vi "PH_PSDBController.ProcCases.vi"(0 "i ref in":refnum<vi>, 1 "selector":string, 2 "Data":T1, 3 "call cluster":T2={"Object"="", "Selector"="", "CallType"=enum."synchronous", "Async Object"="", "Async Selector"="", "Data Descriptor"="", "Data"=[], "Error #"=0, "Expire"=0}, 5 "error in":errorcluster) -> (14 "i ref out":refnum<vi>, 17 "answer cluster":T2={"Object"="", "Selector"="", "CallType"=enum."synchronous", "Async Object"="", "Async Selector"="", "Data Descriptor"="", "Data"=[], "Error #"=0, "Expire"=0}, 19 "error out":errorcluster)   [LabVIEW 2014, in "PH_PSDBController.lvlib"]
doc: "This method is called by a process from within the default case in the event loop. The methods of a class that are linked to events will be called from THIS method. Add your code here."
uses:
  PH_PSDBController.lvlib
  CSCore/CSSystem/CoreDefs/CoreDefs.call_type.ctl
  CSCore/BaseProcess/BaseProcess.descriptor string definition.ctl
  CSCore/CSSystem/CoreDefs/CoreDefs.rawDataType.ctl
  PH_PSDBWriter/PH_PSDBWriter.Data Status.ctl
  PH_Beamline_Chief/PH_Beamline_Chief.Section.ctl
  PH_PSDBWriter/PH_PSDBWriter.PHELIX-Subsystems.ctl
  CSCore/CSSystem/CoreLib/CoreLib.string 2 byte array.vi
  CSCore/CSSystem/CoreLib/CoreLib.byte array 2 short.vi
  CSCore/CSSystem/CoreLib/CoreLib.byte array 2 string.vi
  CSCore/BaseProcess/BaseProcess.lvlib
  CSCore/CSSystem/CoreLib/CoreLib.lvlib
  CSCore/CAEObj/CAEObj.lvlib
  PH_PSDBWriter/PH_PSDBWriter.lvlib
  PH_Common/PH_Common.lvlib
  lib.lib/DimLVEvent/LVDimInterface/LVDimInterface.lvlib
  lib.lib/UtilityLib/UtilityLib.lvlib
  PH_Beamline_Chief/PH_Beamline_Chief.lvlib
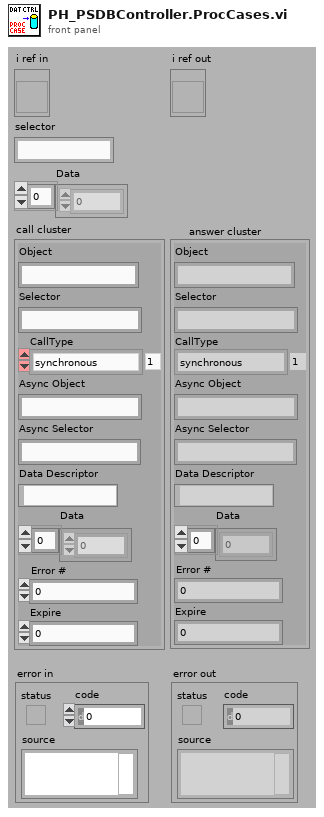
[diagram p1: front panel]
types:
  T1 = typedef "CoreDefs.rawDataType.ctl" = i8[]
  T2 = typedef "CoreDefs.call_type.ctl" = cluster{"Object":string, "Selector":string, "CallType":enum16{"simple", "synchronous", "asynchronous"}, "Async Object":string, "Async Selector":string, "Data Descriptor":T3, "Data":T1, "Error #":i32, "Expire":u32}
  T3 = typedef "BaseProcess.lvlib/BaseProcess.descriptor string definition.ctl" = string
  T4 = typedef "PH_PSDBWriter.lvlib/PH_PSDBWriter.Data Status.ctl" = i16
  T5 = typedef "PH_PSDBController.lvlib/PH_PSDBController.i attribute.ctl" = cluster{"GUI Refs":cluster{"Data Status":refnum<vi>, "Current Shot ID":refnum<vi>, "active Subsystems":refnum<vi>, "Experiment Description":refnum<vi>, "Shot Comment":refnum<vi>, "Experiment":refnum<vi>, "Shottype":refnum<vi>, "Sequencer SM State":refnum<vi>, "Instances with Errors":refnum<vi>}, "Service ID Shot ID":i32, "Service ID wanted Subsystem":i32, "Data Status":T4, "Shotinformation":cluster{"Current Experiment ID":i32, "Current Shot Type":i32, "Current Comment":string}, "Data taking?":bool, "Service ID current Shottype":i32, "Service ID current Experiment":i32, "Service ID currentShot Comment":i32, "Service ID possible Shottypes":i32, "Service ID possible Experiments":i32, "possible Experiments":T6[], "possible Shottypes":T6[], "List":cluster{"Info":cluster{"Instance":string, "Data Status":T4}[], "GUI Ref":refnum<vi>, "Classname":string}[], "Subsystems Off?":cluster{"PHELIX_Beamline_fs_YLF_BL_Status":bool, "PHELIX_Beamline_ns_BL_Status":bool, "PHELIX_Beamline_PA_Input_BL_Status":bool, "PHELIX_Beamline_PA_MA_BL_Status":bool, "PHELIX_Beamline_MA_Z6_BL_Status":bool, "PHELIX_Beamline_MA_LB_BL_Status":bool, "PHELIX_Beamline_PA_LL_BL_Status":bool}, "PSDB Credentials":T7}
  T6 = typedef "PSDB.lvlib/PSDB_Info.ctl" = cluster{"Name":string, "Description":string, "ID":i32}
  T7 = typedef "PH_Common.lvlib/PH_Connection.PSDB Credentials.ctl" = cluster{"PW":string, "ID":string, "DS":string}
  T8 = typedef "PH_Beamline_Chief.lvlib/PH_Beamline_Chief.Section.ctl" = enum16{"None", "YLF", "fs", "fs-YLF", "ns", "PA-Input", "PA-Undelay", "PA-Delay", "PA-before-Bypass", "PA", "PA-Bypass", "PA-Exit", "PA-LL", "LL", "PA-MA", "MA-Exit", "MA-Z6", "Z6", "MA-LB", "LB-TB2", "LB-TB3"}
  T9 = typedef "PH_PSDBWriter.lvlib/PH_PSDBWriter.PHELIX-Subsystems.ctl" = i32
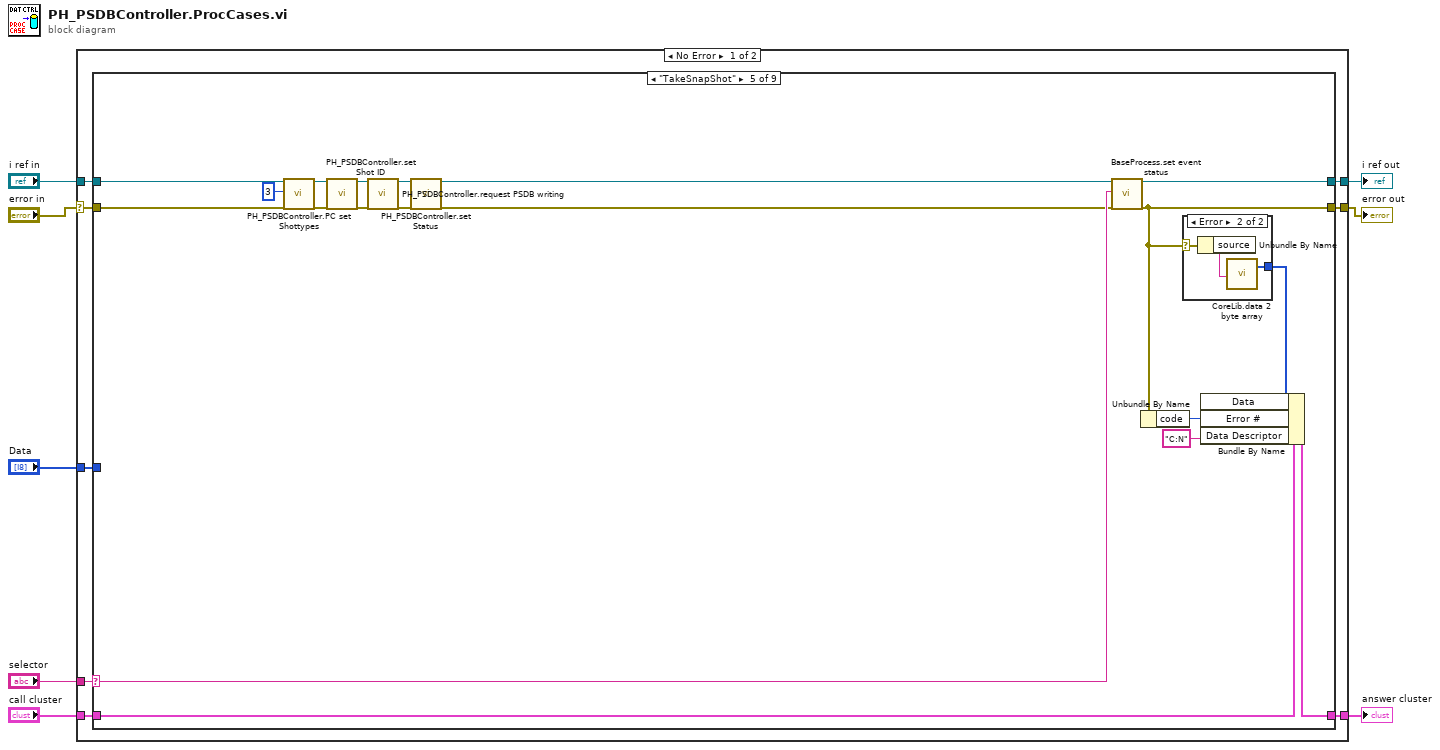
[diagram p0: block diagram]
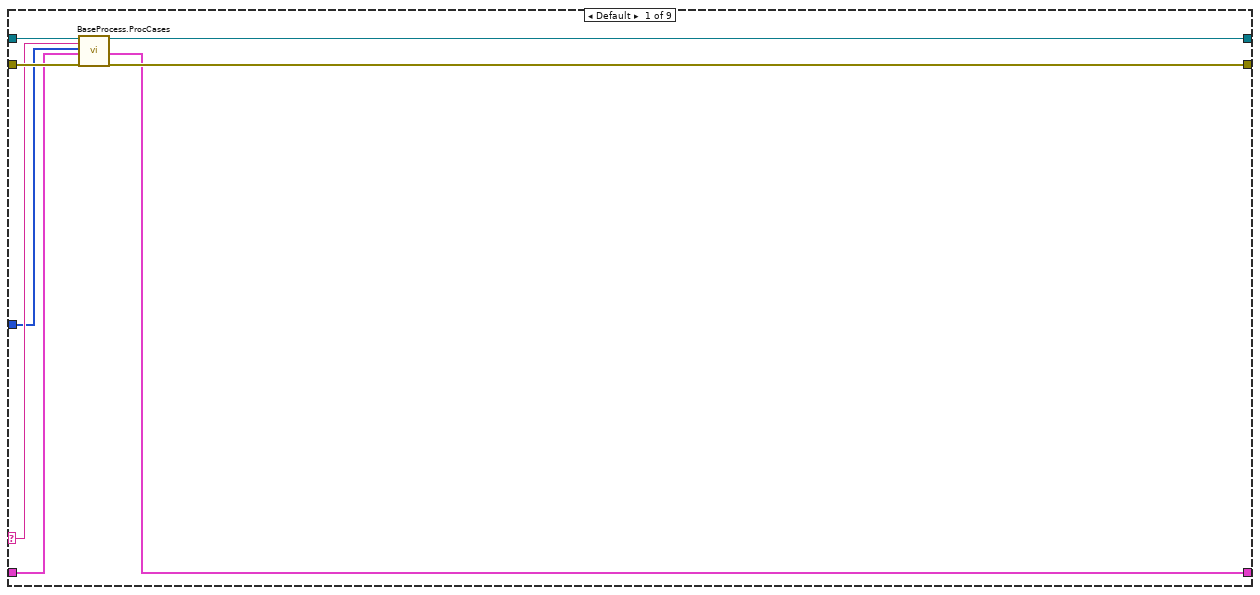
[diagram p2: hidden frame]
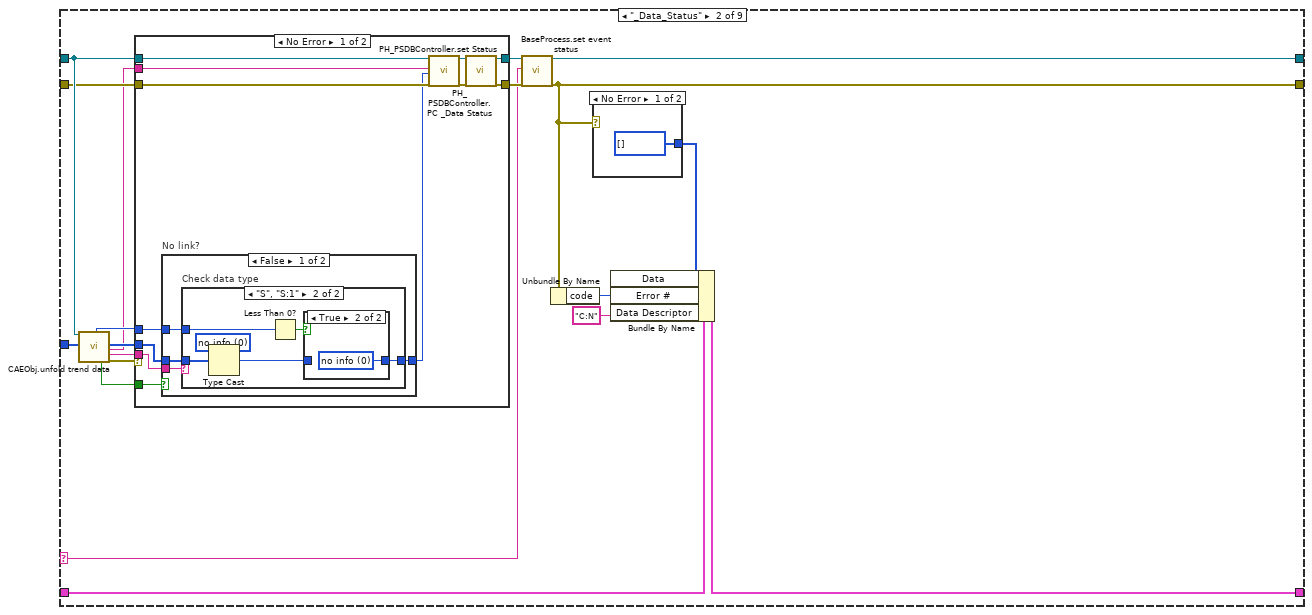
[diagram p3: hidden frame]
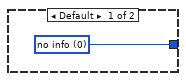
[diagram p4: hidden frame]
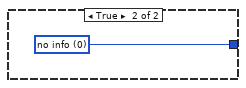
[diagram p6: hidden frame]
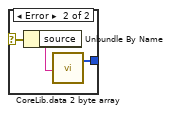
[diagram p8: hidden frame]
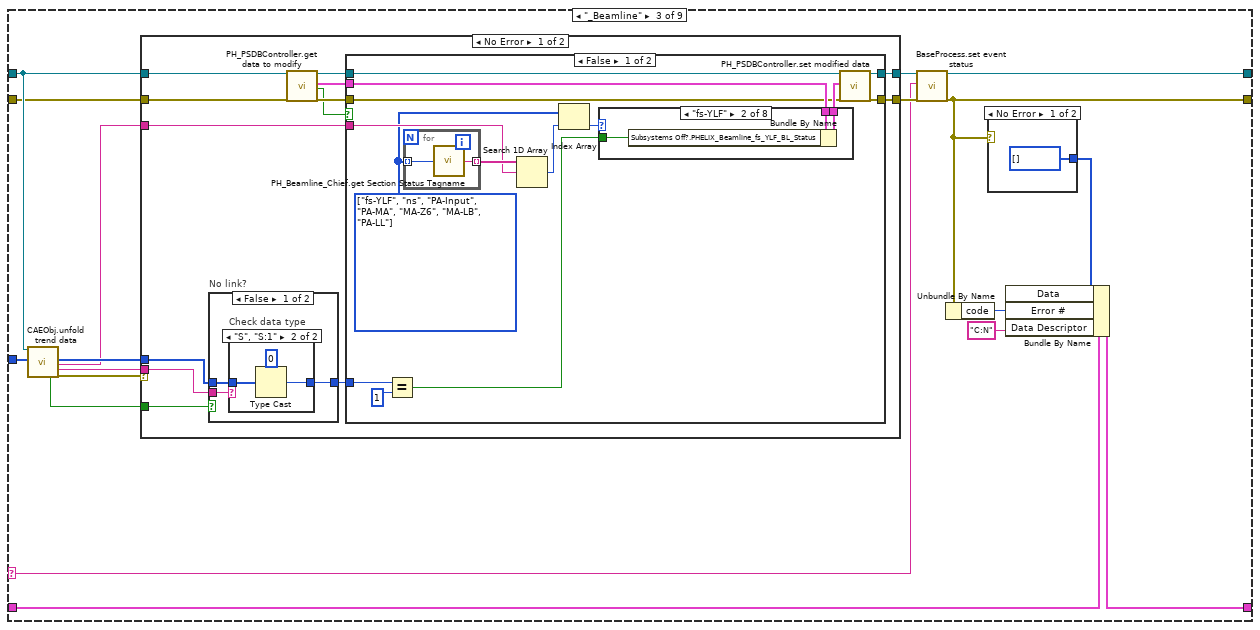
[diagram p9: hidden frame]
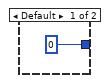
[diagram p10: hidden frame]
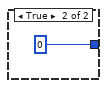
[diagram p11: hidden frame]
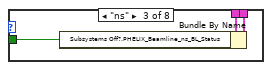
[diagram p13: hidden frame]
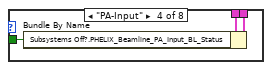
[diagram p14: hidden frame]
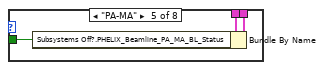
[diagram p15: hidden frame]
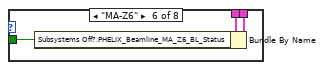
[diagram p16: hidden frame]
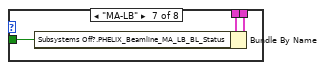
[diagram p17: hidden frame]
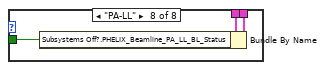
[diagram p18: hidden frame]
diagram:
  n1 = case shown="No Error" "error in" {
    selector: "error in" -> [w9 w435]
    tunnel: "selector" -> [w16 _]
    tunnel: [w15 w434] -> w7
    tunnel: "call cluster" -> [w14 w434]
    tunnel: "i ref in" -> [w13 w436]
    tunnel: [w12 w436] -> w4
    tunnel: [w11 w435] -> w3
    tunnel: "Data" -> [w10 _]
    frame No Error {
      n2 = case shown="\"TakeSnapShot\"" w16 {
        selector: w16 -> [w19 w33 w87 w168 w294 w302 w332 w366 w380]
        tunnel: w10 -> [w17 w26 w80 w161 _ _ _ _ _]
        tunnel: w13 -> [w18 w32 w86 w167 w280 w309 w339 w368 w387]
        tunnel: [w24 w31 w85 w166 w293 w313 w343 w372 w391] -> w12
        tunnel: w14 -> [w20 w28 w82 w163 w290 w306 w336 w367 w384]
        tunnel: [w21 w29 w83 w164 w291 w311 w341 w370 w389] -> w15
        tunnel: w9 -> [w23 w27 w81 w162 w279 w310 w340 w369 w388]
        tunnel: [w22 w30 w84 w165 w292 w312 w342 w371 w390] -> w11
        frame Default {
          n3 = call "BaseProcess.ProcCases.vi"("i ref in"=w18, "selector"=w19, "Data"=w17, "call cluster"=w20, "error in (no error)"=w23) -> ("i ref out"=w24:refnum<vi>, "answer cluster"=w21:T2, "error out"=w22:errorcluster)  [unwired: 12 in]
        }
        frame "_Data_Status" {
          n4 = call "CAEObj.unfold trend data.vi"("i ref in"=w32, "raw trend data"=w26) -> ("quality"=w34:i32, "no link"=w37:bool, "data"=w35:i8[], "serviceName"=w25:string, "typeDescriptor"=w36:string, "error out"=w38:errorcluster)  [unwired: 9 in, 3 out]
          n5 = case shown="No Error" w38 {
            tunnel: w27 -> [w54 w71]
            tunnel: [w46 w70] -> w40
            tunnel: [w44 w71] -> w39
            tunnel: w32 -> [w55 w70]
            tunnel: w37 -> [w51 _]
            tunnel: w36 -> [w52 _]
            tunnel: w35 -> [w50 _]
            tunnel: w34 -> [w49 _]
            tunnel: w25 -> [w53 _]
            frame No Error {
              n6 = case "No link?" shown="False" w51 {
                tunnel: [w59 w69] -> w48
                tunnel: w49 -> [w58 _]
                tunnel: w50 -> [w57 _]
                tunnel: w52 -> [w56 _]
                frame False {
                  n7 = case "Check data type" shown="\"S\", \"S:1\"" w56 {
                    tunnel: [w60 w66] -> w59
                    tunnel: w58 -> [_ w64]
                    tunnel: w57 -> [_ w63]
                    frame Default {
                      w60 = T4 0 items=["no info", "no Data collection", "no problem", "Error getting the instance ID", "Error writing Data to data base", "Error concerning the subsystem"] ("Data Status")
                    }
                    frame "S", "S:1" {
                      w61 = T4 0 items=["no info", "no Data collection", "no problem", "Error getting the instance ID", "Error writing Data to data base", "Error concerning the subsystem"] ("Data Status")
                      n8 = Type Cast(type=w61, x=w63) -> (*(type *) &x=w62:T4)
                      n9 = Less Than 0?(x=w64) -> (x < 0?=w65:bool)
                      n10 = case shown="True" w65 {
                        tunnel: [w67 w68] -> w66
                        tunnel: w62 -> [w67 _]
                        frame False {
                        }
                        frame True {
                          w68 = T4 0 items=["no info", "no Data collection", "no problem", "Error getting the instance ID", "Error writing Data to data base", "Error concerning the subsystem"] ("Data Status")
                        }
                      }
                    }
                  }
                }
                frame True {
                  w69 = T4 0 items=["no info", "no Data collection", "no problem", "Error getting the instance ID", "Error writing Data to data base", "Error concerning the subsystem"] ("Data Status")
                }
              }
              n11 = call "PH_PSDBController.PC _Data Status.vi"("i ref in"=w55, "Data Status service name"=w53, "Data Status"=w48, "error IO"=w54) -> ("i ref out"=w47:refnum<vi>, "error out"=w45:errorcluster)  [unwired: 14 in]
              n12 = call "PH_PSDBController.set Status.vi"("i ref in"=w47, "error in"=w45) -> ("i ref out"=w46:refnum<vi>, "error out"=w44:errorcluster)  [unwired: 16 in]
            }
            frame Error {
            }
          }
          n13 = call "BaseProcess.set event status.vi"("i ref in"=w40, "EventStatus"=w33, "error in (no error)"=w39) -> ("i ref out"=w31:refnum<vi>, "error out"=w30:errorcluster)  [unwired: 14 in, 1 out]
          n14 = Unbundle By Name(w30) -> ("code"=w43:i32)
          n15 = case shown="No Error" w30 {
            selector: w30 -> [_ w75]
            tunnel: [T1 [] ("byteArray out") w73] -> w41
            frame No Error {
            }
            frame Error {
              n16 = Unbundle By Name(w75) -> ("source"=w74:string)
              n17 = call-poly "CoreLib.data 2 byte array.vi"("string"=w74) -> ("byteArray out"=w73:T1)  [unwired: 18 in]
            }
          }
          n18 = Bundle By Name(cluster=w28, "Data"=w41, "Error #"=w43, "Data Descriptor"="C:N") -> (w29:T2)
        }
        frame "_Beamline" {
          n19 = call "CAEObj.unfold trend data.vi"("i ref in"=w86, "raw trend data"=w80) -> ("no link"=w88:bool, "data"=w78:i8[], "serviceName"=w76:string, "typeDescriptor"=w77:string, "error out"=w79:errorcluster)  [unwired: 9 in, 4 out]
          n20 = case shown="No Error" w79 {
            tunnel: w81 -> [w106 w156]
            tunnel: [w103 w155] -> w90
            tunnel: [w102 w156] -> w89
            tunnel: w86 -> [w105 w155]
            tunnel: w88 -> [w97 _]
            tunnel: w78 -> [w98 _]
            tunnel: w77 -> [w96 _]
            tunnel: w76 -> [w95 _]
            frame No Error {
              n21 = case "No link?" shown="False" w97 {
                tunnel: [w109 i16 0] -> w94
                tunnel: w98 -> [w108 _]
                tunnel: w96 -> [w107 _]
                frame False {
                  n22 = case "Check data type" shown="\"S\", \"S:1\"" w107 {
                    tunnel: [i16 0 w111] -> w109
                    tunnel: w108 -> [_ w112]
                    frame Default {
                    }
                    frame "S", "S:1" {
                      n23 = Type Cast(type=i16 0, x=w112) -> (*(type *) &x=w111:i16)
                    }
                  }
                }
                frame True {
                }
              }
              n24 = call "PH_PSDBController.get data to modify.vi"("i ref in"=w105, "error in (no error)"=w106) -> ("i ref out"=w104:refnum<vi>, "i attribute"=w99:T5, "timed out"=w100:bool, "error out"=w101:errorcluster)  [unwired: 14 in]
              n25 = case shown="False" w100 {
                tunnel: w104 -> [w128 w154]
                tunnel: [w127 w154] -> w103
                tunnel: [w126 w153] -> w102
                tunnel: w101 -> [w120 w153]
                tunnel: w99 -> [w123 _]
                tunnel: w95 -> [w118 _]
                tunnel: w94 -> [w125 _]
                frame False {
                  w115 = T8[] [enum."fs-YLF", enum."ns", enum."PA-Input", enum."PA-MA", enum."MA-Z6", enum."MA-LB", enum."PA-LL"] items=["None", "YLF", "fs", "fs-YLF", "ns", "PA-Input", "PA-Undelay", "PA-Delay", "PA-before-Bypass", "PA", "PA-Bypass", "PA-Exit", "PA-LL", "LL", "PA-MA", "MA-Exit", "MA-Z6", "Z6", "MA-LB", "LB-TB2", "LB-TB3"]
                  n26 = Equal?(x=w125, y=i16 1) -> (x = y?=w122:bool)
                  n27 = for {
                    tunnel: w115 -> [w130] mode=indexing
                    tunnel: [w129] -> w119 mode=indexing
                    n28 = call "PH_Beamline_Chief.get Section Status Tagname.vi"("Beamline Section"=w130) -> ("Section Status Tagname"=w129:string)
                  }
                  n29 = Search 1D Array(1D array=w119, element=w118) -> (index of element=w117:i32)  [unwired: 1 in]
                  n30 = Index Array(array=w115, index=w117) -> (element=w116:T8)
                  n31 = case shown="\"fs-YLF\"" w116 {
                    tunnel: w123 -> [w131 w134 w137 w140 w143 w146 w149 w152]
                    tunnel: [w131 w133 w136 w139 w142 w145 w148 w151] -> w121
                    tunnel: w122 -> [_ w132 w135 w138 w141 w144 w147 w150]
                    frame Default {
                    }
                    frame "fs-YLF" {
                      n32 = Bundle By Name(cluster=w134, "Subsystems Off?.PHELIX_Beamline_fs_YLF_BL_Status"=w132) -> (w133:T5)
                    }
                    frame "ns" {
                      n33 = Bundle By Name(cluster=w137, "Subsystems Off?.PHELIX_Beamline_ns_BL_Status"=w135) -> (w136:T5)
                    }
                    frame "PA-Input" {
                      n34 = Bundle By Name(cluster=w140, "Subsystems Off?.PHELIX_Beamline_PA_Input_BL_Status"=w138) -> (w139:T5)
                    }
                    frame "PA-MA" {
                      n35 = Bundle By Name(cluster=w143, "Subsystems Off?.PHELIX_Beamline_PA_MA_BL_Status"=w141) -> (w142:T5)
                    }
                    frame "MA-Z6" {
                      n36 = Bundle By Name(cluster=w146, "Subsystems Off?.PHELIX_Beamline_MA_Z6_BL_Status"=w144) -> (w145:T5)
                    }
                    frame "MA-LB" {
                      n37 = Bundle By Name(cluster=w149, "Subsystems Off?.PHELIX_Beamline_MA_LB_BL_Status"=w147) -> (w148:T5)
                    }
                    frame "PA-LL" {
                      n38 = Bundle By Name(cluster=w152, "Subsystems Off?.PHELIX_Beamline_PA_LL_BL_Status"=w150) -> (w151:T5)
                    }
                  }
                  n39 = call "PH_PSDBController.set modified data.vi"("i ref in"=w128, "i attribute"=w121, "error in (no error)"=w120) -> ("i ref out"=w127:refnum<vi>, "error out"=w126:errorcluster)  [unwired: 15 in]
                }
                frame True {
                }
              }
            }
            frame Error {
            }
          }
          n40 = call "BaseProcess.set event status.vi"("i ref in"=w90, "EventStatus"=w87, "error in (no error)"=w89) -> ("i ref out"=w85:refnum<vi>, "error out"=w84:errorcluster)  [unwired: 14 in, 1 out]
          n41 = Unbundle By Name(w84) -> ("code"=w93:i32)
          n42 = case shown="No Error" w84 {
            selector: w84 -> [_ w160]
            tunnel: [T1 [] ("byteArray out") w158] -> w91
            frame No Error {
            }
            frame Error {
              n43 = Unbundle By Name(w160) -> ("source"=w159:string)
              n44 = call-poly "CoreLib.data 2 byte array.vi"("string"=w159) -> ("byteArray out"=w158:T1)  [unwired: 18 in]
            }
          }
          n45 = Bundle By Name(cluster=w82, "Data"=w91, "Error #"=w93, "Data Descriptor"="C:N") -> (w83:T2)
        }
        frame "_Sequencer_State" {
          n46 = call "CAEObj.unfold trend data.vi"("i ref in"=w167, "raw trend data"=w161) -> ("quality"=w169:i32, "no link"=w172:bool, "data"=w170:i8[], "typeDescriptor"=w171:string, "error out"=w173:errorcluster)  [unwired: 9 in, 4 out]
          n47 = case shown="No Error" w173 {
            tunnel: w162 -> [w193 w274]
            tunnel: [w196 w273] -> w175
            tunnel: [w197 w274] -> w174
            tunnel: w167 -> [w191 w273]
            tunnel: w172 -> [w188 _]
            tunnel: w171 -> [w198 _]
            tunnel: w170 -> [w199 _]
            tunnel: w169 -> [w200 _]
            frame No Error {
              n48 = call "PH_PSDBController.get i attribute.vi"("i ref in"=w191, "error in (no error)"=w193) -> ("i ref out"=w190:refnum<vi>, "i attribute"=w186:T5, "error out"=w192:errorcluster)  [unwired: 15 in]
              n49 = call "PH_DIM.get String.vi"("no link"=w188, "typeDescriptor"=w198, "data"=w199, "quality"=w200) -> ("Output String"=w195:string)
              n50 = Unbundle By Name(w186) -> ("Subsystems Off?.PHELIX_Beamline_fs_YLF_BL_Status"=w179:bool, "Subsystems Off?.PHELIX_Beamline_ns_BL_Status"=w180:bool, "Subsystems Off?.PHELIX_Beamline_PA_Input_BL_Status"=w181:bool, "Subsystems Off?.PHELIX_Beamline_PA_MA_BL_Status"=w182:bool, "Subsystems Off?.PHELIX_Beamline_MA_Z6_BL_Status"=w183:bool, "Subsystems Off?.PHELIX_Beamline_MA_LB_BL_Status"=w184:bool, "Subsystems Off?.PHELIX_Beamline_PA_LL_BL_Status"=w185:bool, "GUI Refs.Sequencer SM State"=w187:refnum<vi>)
              n51 = call "PH_Strings.Remove trailing Zeros.vi"("Input String"=w195) -> ("Output String"=w189:string)
              n52 = call "PH_GUI.set string GUI object.vi"("GUI object Ref"=w187, "Text"=w189, "Blinking? (false)"=w188, "error in"=w192) -> ("error out"=w194:errorcluster)  [unwired: 15 in]
              n53 = case shown="\"Stand by\"" w189 {
                tunnel: w190 -> [w202 w208 w219]
                tunnel: [w201 w207 w224] -> w197
                tunnel: [w202 w206 w223] -> w196
                tunnel: w194 -> [w201 w205 w220]
                tunnel: w185 -> [_ _ w217]
                tunnel: w184 -> [_ _ w215]
                tunnel: w183 -> [_ _ w214]
                tunnel: w182 -> [_ _ w213]
                tunnel: w181 -> [_ _ w212]
                tunnel: w180 -> [_ _ w211]
                tunnel: w179 -> [_ _ w210]
                frame Default {
                }
                frame "Start Slow Devices" {
                  n54 = call "PH_PSDBController.set Shot ID.vi"("i ref in"=w208, "error in"=w205) -> ("i ref out"=w203:refnum<vi>, "error out"=w204:errorcluster)  [unwired: 16 in]
                  n55 = call "PH_PSDBController.set Status.vi"("i ref in"=w203, "error in"=w204) -> ("i ref out"=w206:refnum<vi>, "error out"=w207:errorcluster)  [unwired: 16 in]
                }
                frame "Stand by" {
                  n56 = Build Array(w210, w211, w212, w213, w214, w215, w217) -> (w216:bool[])
                  n57 = flat-sequence {
                    tunnel: w216 -> [w226]
                    tunnel: [w226] -> w209
                    tunnel: [w228] -> w218
                    tunnel: w209 -> [w227]
                    frame #0 {
                      n58 = Wait (ms)(milliseconds to wait=u32 1000) -> ()  [unwired: 1 out]
                    }
                    frame #1 {
                      w232 = T9[] [0, 11, 12, 1, 2, 3, 4, 5, 7, 10, 8, 6, 9] items=["Miscellaneous", "fs-Frontend", "ns-Frontend", "PreAmp", "MainAmp", "MAS", "COS", "Beamline", "Experiment Laserbay", "Experiment Laserlabor", "Experiment Z6", "Timing", "Pulsed Power"] ("Wanted Subsystems")
                      n59 = Array Subset(array=w232, index=0, length=3) -> (w231:T9[])
                      n60 = for {
                        tunnel: w227 -> [w235] mode=indexing
                        shift-right: [w237] -> w228
                        shift-left: w231 -> [w236]
                        tunnel: w232 -> [w234]
                        i -> [w233]
                        n61 = case shown="False" w235 {
                          tunnel: [w242 w272] -> w237
                          tunnel: w236 -> [w241 w272]
                          tunnel: w234 -> [w240 _]
                          tunnel: w233 -> [w238 _]
                          frame False {
                            n62 = case shown="Default" w238 {
                              tunnel: w240 -> [_ w247 w251 w255 w259 w263 w267 w271]
                              tunnel: [w243 w246 w250 w254 w258 w262 w266 w270] -> w239
                              frame Default {
                                w243 = T9[] [] items=["Miscellaneous", "fs-Frontend", "ns-Frontend", "PreAmp", "MainAmp", "MAS", "COS", "Beamline", "Experiment Laserbay", "Experiment Laserlabor", "Experiment Z6", "Timing", "Pulsed Power"]
                              }
                              frame 0 {
                                n63 = Array Subset(array=w247, index=3, length=1) -> (w246:T9[])
                              }
                              frame 1 {
                                n64 = Array Subset(array=w251, index=4, length=1) -> (w250:T9[])
                              }
                              frame 2 {
                                n65 = Array Subset(array=w255, index=5, length=1) -> (w254:T9[])
                              }
                              frame 3 {
                                n66 = Array Subset(array=w259, index=6, length=3) -> (w258:T9[])
                              }
                              frame 4 {
                                n67 = Array Subset(array=w263, index=9, length=1) -> (w262:T9[])
                              }
                              frame 5 {
                                n68 = Array Subset(array=w267, index=10, length=2) -> (w266:T9[])
                              }
                              frame 6 {
                                n69 = Array Subset(array=w271, index=12, length=1) -> (w270:T9[])
                              }
                            }
                            n70 = Insert Into Array(array=w241, new element=w239) -> (w242:T9[])  [unwired: 1 in]
                          }
                          frame True {
                          }
                        }
                      }
                    }
                  }
                  n71 = call "PH_PSDBController.request PSDB writing.vi"("i ref in"=w219, "Wanted Subsystems"=w218, "error IO"=w220) -> ("i ref out"=w222:refnum<vi>, "error out"=w221:errorcluster)  [unwired: 15 in]
                  n72 = call "PH_PSDBController.set Status.vi"("i ref in"=w222, "error in"=w221) -> ("i ref out"=w223:refnum<vi>, "error out"=w224:errorcluster)  [unwired: 16 in]
                }
              }
            }
            frame Error {
            }
          }
          n73 = call "BaseProcess.set event status.vi"("i ref in"=w175, "EventStatus"=w168, "error in (no error)"=w174) -> ("i ref out"=w166:refnum<vi>, "error out"=w165:errorcluster)  [unwired: 14 in, 1 out]
          n74 = Unbundle By Name(w165) -> ("code"=w178:i32)
          n75 = case shown="Error" w165 {
            selector: w165 -> [_ w278]
            tunnel: [T1 [] ("byteArray out") w276] -> w176
            frame No Error {
            }
            frame Error {
              n76 = Unbundle By Name(w278) -> ("source"=w277:string)
              n77 = call-poly "CoreLib.data 2 byte array.vi"("string"=w277) -> ("byteArray out"=w276:T1)  [unwired: 18 in]
            }
          }
          n78 = Bundle By Name(cluster=w163, "Data"=w176, "Error #"=w178, "Data Descriptor"="C:N") -> (w164:T2)
        }
        frame "TakeSnapShot" {
          n79 = call "PH_PSDBController.PC set Shottypes.vi"("i ref in"=w280, "Shottype"=i16 3, "error IO"=w279) -> ("i ref out"=w285:refnum<vi>, "error out"=w284:errorcluster)  [unwired: 15 in]
          n80 = call "PH_PSDBController.set Shot ID.vi"("i ref in"=w285, "error in"=w284) -> ("i ref out"=w282:refnum<vi>, "error out"=w281:errorcluster)  [unwired: 16 in]
          n81 = call "PH_PSDBController.request PSDB writing.vi"("i ref in"=w282, "error IO"=w281) -> ("i ref out"=w286:refnum<vi>, "error out"=w289:errorcluster)  [unwired: 16 in]
          n82 = call "PH_PSDBController.set Status.vi"("i ref in"=w286, "error in"=w289) -> ("i ref out"=w287:refnum<vi>, "error out"=w288:errorcluster)  [unwired: 16 in]
          n83 = call "BaseProcess.set event status.vi"("i ref in"=w287, "EventStatus"=w294, "error in (no error)"=w288) -> ("i ref out"=w293:refnum<vi>, "error out"=w292:errorcluster)  [unwired: 14 in, 1 out]
          n84 = Unbundle By Name(w292) -> ("code"=w297:i32)
          n85 = case shown="Error" w292 {
            selector: w292 -> [_ w301]
            tunnel: [T1 [] ("byteArray out") w299] -> w295
            frame No Error {
            }
            frame Error {
              n86 = Unbundle By Name(w301) -> ("source"=w300:string)
              n87 = call-poly "CoreLib.data 2 byte array.vi"("string"=w300) -> ("byteArray out"=w299:T1)  [unwired: 18 in]
            }
          }
          n88 = Bundle By Name(cluster=w290, "Data"=w295, "Error #"=w297, "Data Descriptor"="C:N") -> (w291:T2)
        }
        frame "SetShotType" {
          n89 = Unbundle By Name(w306) -> ("Data"=w305:T1)
          n90 = call-poly "CoreLib.byte array 2 data.vi"("byteArray"=w305) -> ("i16"=w304:i16, "error out"=w303:errorcluster)  [unwired: 16 in, 1 out]
          n91 = case shown="No Error" w303 {
            tunnel: w310 -> [w323 w327]
            tunnel: w309 -> [w322 w325]
            tunnel: [w319 w325] -> w308
            tunnel: [w317 w326] -> w307
            tunnel: w304 -> [w321 _]
            tunnel: w302 -> [_ w324]
            frame No Error {
              n92 = call "PH_PSDBController.PC set Shottypes.vi"("i ref in"=w322, "Shottype"=w321, "error IO"=w323) -> ("i ref out"=w320:refnum<vi>, "error out"=w318:errorcluster)  [unwired: 15 in]
              n93 = call "PH_PSDBController.set Status.vi"("i ref in"=w320, "error in"=w318) -> ("i ref out"=w319:refnum<vi>, "error out"=w317:errorcluster)  [unwired: 16 in]
            }
            frame Error {
              n94 = call "CoreLib.set data type mismatch.vi"("error in (no error)"=w327, "error source"=w324) -> ("error out"=w326:errorcluster)  [unwired: 17 in]
            }
          }
          n95 = call "BaseProcess.set event status.vi"("i ref in"=w308, "EventStatus"=w302, "error in (no error)"=w307) -> ("i ref out"=w313:refnum<vi>, "error out"=w312:errorcluster)  [unwired: 14 in, 1 out]
          n96 = Unbundle By Name(w312) -> ("code"=w316:i32)
          n97 = case shown="Error" w312 {
            selector: w312 -> [_ w331]
            tunnel: [T1 [] ("byteArray out") w329] -> w314
            frame No Error {
            }
            frame Error {
              n98 = Unbundle By Name(w331) -> ("source"=w330:string)
              n99 = call-poly "CoreLib.data 2 byte array.vi"("string"=w330) -> ("byteArray out"=w329:T1)  [unwired: 18 in]
            }
          }
          n100 = Bundle By Name(cluster=w306, "Data"=w314, "Error #"=w316, "Data Descriptor"="C:N") -> (w311:T2)
        }
        frame "SetExpID" {
          n101 = Unbundle By Name(w336) -> ("Data"=w335:T1)
          n102 = call-poly "CoreLib.byte array 2 data.vi"("byteArray"=w335) -> ("i16"=w334:i16, "error out"=w333:errorcluster)  [unwired: 16 in, 1 out]
          n103 = case shown="No Error" w333 {
            tunnel: w340 -> [w353 w357]
            tunnel: w339 -> [w352 w355]
            tunnel: [w349 w355] -> w338
            tunnel: [w347 w356] -> w337
            tunnel: w334 -> [w351 _]
            tunnel: w332 -> [_ w354]
            frame No Error {
              n104 = call "PH_PSDBController.PC set Exp ID.vi"("i ref in"=w352, "Exp ID"=w351, "error IO"=w353) -> ("i ref out"=w350:refnum<vi>, "error out"=w348:errorcluster)  [unwired: 15 in]
              n105 = call "PH_PSDBController.set Status.vi"("i ref in"=w350, "error in"=w348) -> ("i ref out"=w349:refnum<vi>, "error out"=w347:errorcluster)  [unwired: 16 in]
            }
            frame Error {
              n106 = call "CoreLib.set data type mismatch.vi"("error in (no error)"=w357, "error source"=w354) -> ("error out"=w356:errorcluster)  [unwired: 17 in]
            }
          }
          n107 = call "BaseProcess.set event status.vi"("i ref in"=w338, "EventStatus"=w332, "error in (no error)"=w337) -> ("i ref out"=w343:refnum<vi>, "error out"=w342:errorcluster)  [unwired: 14 in, 1 out]
          n108 = Unbundle By Name(w342) -> ("code"=w346:i32)
          n109 = case shown="Error" w342 {
            selector: w342 -> [_ w361]
            tunnel: [T1 [] ("byteArray out") w359] -> w344
            frame No Error {
            }
            frame Error {
              n110 = Unbundle By Name(w361) -> ("source"=w360:string)
              n111 = call-poly "CoreLib.data 2 byte array.vi"("string"=w360) -> ("byteArray out"=w359:T1)  [unwired: 18 in]
            }
          }
          n112 = Bundle By Name(cluster=w336, "Data"=w344, "Error #"=w346, "Data Descriptor"="C:N") -> (w341:T2)
        }
        frame "GetPSDBInfo" {
          n113 = call "PH_PSDBController.PC get PSDB Information.vi"("i ref in"=w368, "error IO"=w369) -> ("i ref out"=w365:refnum<vi>, "error out"=w363:errorcluster)  [unwired: 16 in]
          n114 = call "PH_PSDBController.set Status.vi"("i ref in"=w365, "error in"=w363) -> ("i ref out"=w364:refnum<vi>, "error out"=w362:errorcluster)  [unwired: 16 in]
          n115 = call "BaseProcess.set event status.vi"("i ref in"=w364, "EventStatus"=w366, "error in (no error)"=w362) -> ("i ref out"=w372:refnum<vi>, "error out"=w371:errorcluster)  [unwired: 14 in, 1 out]
          n116 = Unbundle By Name(w371) -> ("code"=w375:i32)
          n117 = case shown="Error" w371 {
            selector: w371 -> [_ w379]
            tunnel: [T1 [] ("byteArray out") w377] -> w373
            frame No Error {
            }
            frame Error {
              n118 = Unbundle By Name(w379) -> ("source"=w378:string)
              n119 = call-poly "CoreLib.data 2 byte array.vi"("string"=w378) -> ("byteArray out"=w377:T1)  [unwired: 18 in]
            }
          }
          n120 = Bundle By Name(cluster=w367, "Data"=w373, "Error #"=w375, "Data Descriptor"="C:N") -> (w370:T2)
        }
        frame "SetShotComment" {
          n121 = Unbundle By Name(w384) -> ("Data"=w383:T1)
          n122 = call-poly "CoreLib.byte array 2 data.vi"("byteArray"=w383) -> ("string"=w382:string, "error out"=w381:errorcluster)  [unwired: 16 in, 1 out]
          n123 = case shown="No Error" w381 {
            tunnel: w388 -> [w398 w429]
            tunnel: w387 -> [w399 w427]
            tunnel: [w396 w427] -> w386
            tunnel: [w397 w428] -> w385
            tunnel: w382 -> [w395 _]
            tunnel: w380 -> [_ w426]
            frame No Error {
              n124 = call "PH_PSDBController.get data to modify.vi"("i ref in"=w399, "error in (no error)"=w398) -> ("i ref out"=w402:refnum<vi>, "i attribute"=w401:T5, "timed out"=w403:bool, "error out"=w400:errorcluster)  [unwired: 14 in]
              n125 = case shown="False" w403 {
                tunnel: w400 -> [w404 w424]
                tunnel: w401 -> [w408 _]
                tunnel: w395 -> [w405 _]
                tunnel: w402 -> [w412 w425]
                tunnel: [w411 w425] -> w396
                tunnel: [w410 w424] -> w397
                frame False {
                  n126 = Unbundle By Name(w408) -> ("Service ID currentShot Comment"=w413:i32, "GUI Refs.Shot Comment"=w415:refnum<vi>)
                  n127 = call "PH_Strings.Remove trailing Zeros.vi"("Input String"=w405) -> ("Output String"=w406:string)
                  n128 = Bundle By Name(cluster=w408, "Shotinformation.Current Comment"=w406) -> (w407:T5)
                  n129 = call "PH_GUI.set string GUI object.vi"("GUI object Ref"=w415, "Text"=w406, "error in"=w404) -> ("error out"=w414:errorcluster)  [unwired: 16 in]
                  n130 = case shown="Default" w413 {
                    selector: w413 -> [_ w422]
                    tunnel: [w416 w423] -> w409
                    tunnel: w414 -> [w416 w421]
                    tunnel: w405 -> [_ w419]
                    frame -1 {
                    }
                    frame Default {
                      n131 = call "UtilityLib.align string.vi"("stringIn"=w419, "stringLength (80)"=u16 1024, "error in (no error)"=w421) -> ("stringOut"=w418:string, "error out"=w420:errorcluster)  [unwired: 15 in]
                      n132 = call "LVDimInterface.dis_update_service.vi"("my_serviceID"=w422, "data"=w418, "error in (no error)"=w420) -> ("error out"=w423:errorcluster)  [unwired: 14 in, 2 out]
                    }
                  }
                  n133 = call "PH_PSDBController.set modified data.vi"("i ref in"=w412, "i attribute"=w407, "error in (no error)"=w409) -> ("i ref out"=w411:refnum<vi>, "error out"=w410:errorcluster)  [unwired: 15 in]
                }
                frame True {
                }
              }
            }
            frame Error {
              n134 = call "CoreLib.set data type mismatch.vi"("error in (no error)"=w429, "error source"=w426) -> ("error out"=w428:errorcluster)  [unwired: 17 in]
            }
          }
          n135 = call "BaseProcess.set event status.vi"("i ref in"=w386, "EventStatus"=w380, "error in (no error)"=w385) -> ("i ref out"=w391:refnum<vi>, "error out"=w390:errorcluster)  [unwired: 14 in, 1 out]
          n136 = Unbundle By Name(w390) -> ("code"=w394:i32)
          n137 = case shown="Error" w390 {
            selector: w390 -> [_ w433]
            tunnel: [T1 [] ("byteArray out") w431] -> w392
            frame No Error {
            }
            frame Error {
              n138 = Unbundle By Name(w433) -> ("source"=w432:string)
              n139 = call-poly "CoreLib.data 2 byte array.vi"("string"=w432) -> ("byteArray out"=w431:T1)  [unwired: 18 in]
            }
          }
          n140 = Bundle By Name(cluster=w384, "Data"=w392, "Error #"=w394, "Data Descriptor"="C:N") -> (w389:T2)
        }
      }
    }
    frame Error {
    }
  }
  "answer cluster" <- w7
  "i ref out" <- w4
  "error out" <- w3
